vi "Data Analysis.vi"(8 "error in (no error)":errorcluster) -> (0 "error out":errorcluster)   [LabVIEW 2016, in "User Interface.lvlib"]
uses:
  User Interface.lvlib
  DAQ Hardware/Signal name Array.ctl
  DAQ Hardware/Data View Commnd.ctl
  DAQ Hardware/Data Analysis Main Cluster.ctl
  <vilib>/NI/Current Value Table/DataTypes/Array of Double_Read.vi
  <vilib>/NI/Current Value Table/DataTypes/Single_Read.vi
  <vilib>/NI/Current Value Table/DataTypes/Boolean_Read.vi
  <vilib>/NI/Current Value Table/Type to Enum.vi
  <vilib>/NI/Current Value Table/DataTypes/Array of Double_Type To Enum.vi
  <vilib>/NI/Current Value Table/DataTypes/Single_Type To Enum.vi
  <vilib>/NI/Current Value Table/DataTypes/Boolean_Type To Enum.vi
  <vilib>/NI/Current Value Table/FGVs/Group Memory.vi
  <vilib>/NI/Current Value Table/FGVs/Tag Memory.vi
  <vilib>/NI/Current Value Table/FGVs/CVT Globals.vi
  <vilib>/NI/Current Value Table/Memory Block.vi
  <vilib>/NI/Current Value Table/DataTypes/Array of Double_Memory Block.vi
  <vilib>/NI/Current Value Table/DataTypes/Single_Memory Block.vi
  <vilib>/NI/Current Value Table/DataTypes/Boolean_Memory Block.vi
  DAQ Hardware/DAQ Hardware.lvlib
  <vilib>/NI/Current Value Table/Current Value Table.lvlib
panel:
  out "Time":string="Sat  8/3/2019  8:10:44 PM"
  in  "Exit":bool
  out "Analog Data":dbl[][](graph)
  in  "Signal Selection":T1=[{"Select"=FALSE, "Signal name"=""}, {"Select"=FALSE, "Signal name"=""}, {"Select"=FALSE, "Signal name"=""}, {"Select"=FALSE, "Signal name"=""}]
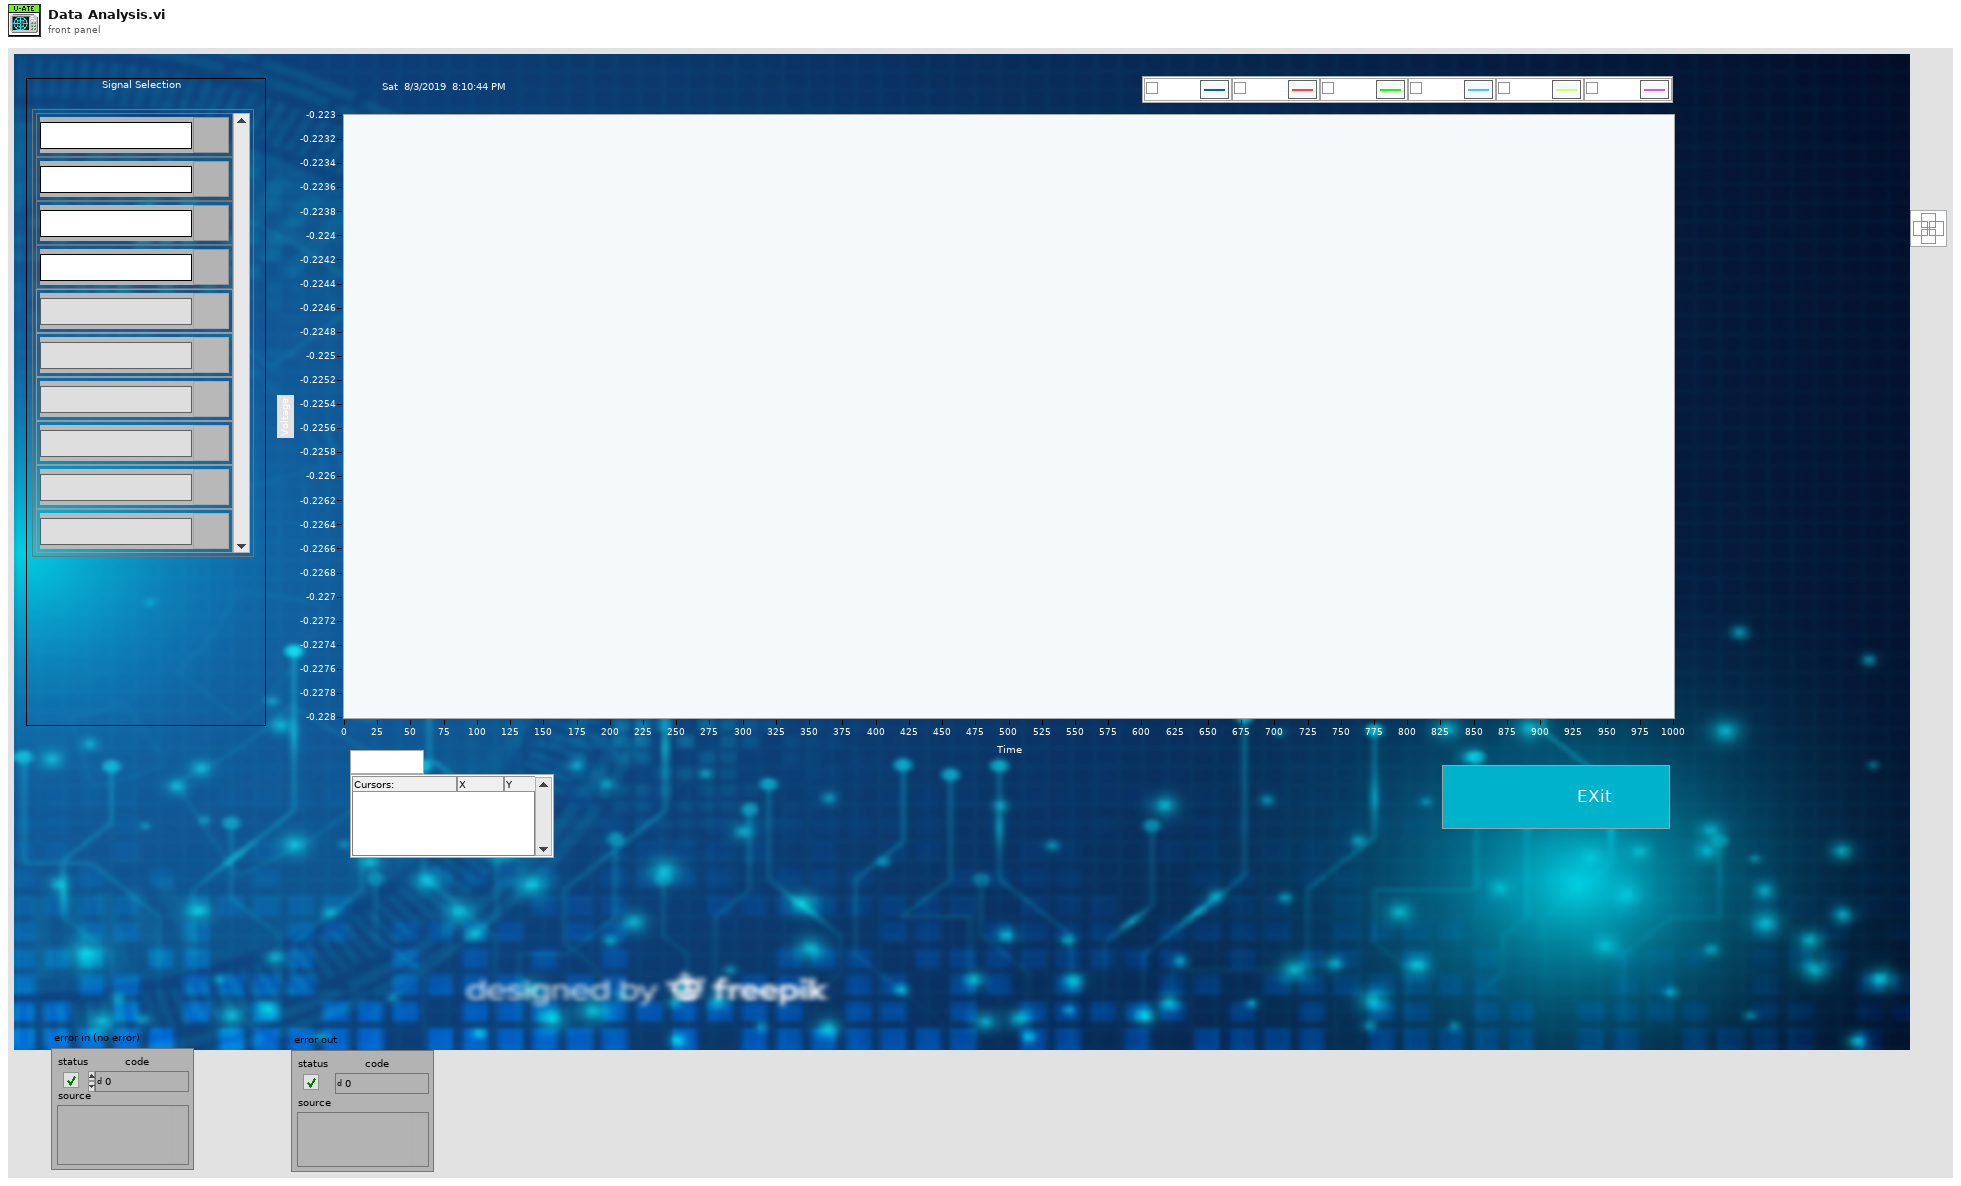
[diagram p1: front panel]
types:
  T1 = typedef "DAQ Hardware.lvlib/Signal name Array.ctl" = cluster{"Select":bool, "Signal name":string}[]
  T2 = typedef "DAQ Hardware.lvlib/Data Analysis Main Cluster.ctl" = cluster{"Active Signal":cluster{"Select":bool, "Signal name":string}[]}
  T3 = typedef "DAQ Hardware.lvlib/Data View Commnd.ctl" = enum16{"Init", "Main", "Close"}
  T4 = typedef "CVT.lvlib/Current Value Table.lvlib/Data Types.ctl" = enum16{"Double", "Single", "I64", "I32", "I16", "I8", "U64", "U32", "U16", "U8", "String", "Boolean", "Array of U8", "Array of U16", "Array of U32", "Array of U64", "Array of I64", "Array of I32", "Array of I16", "Array of I8", "Array of Double", "Array of Single", "Array of Boolean", "Array of String"}
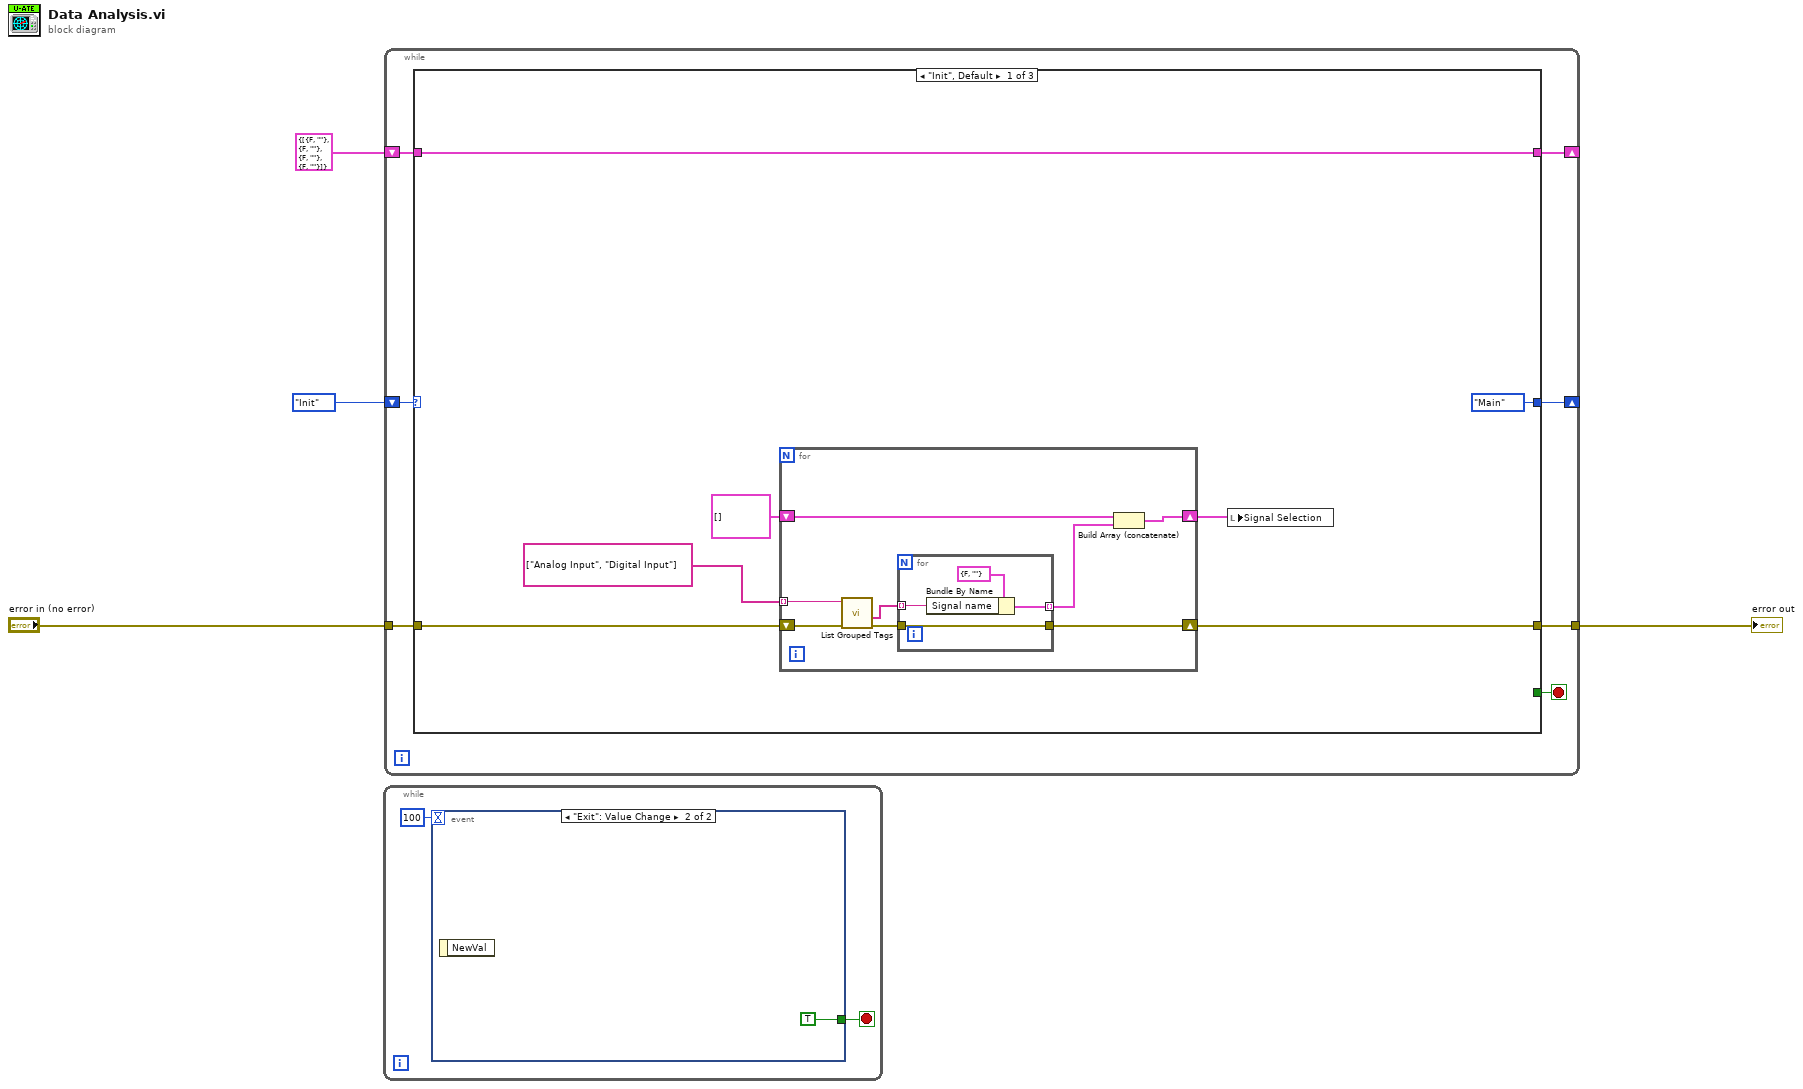
[diagram p0: block diagram]
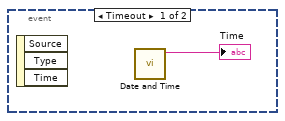
[diagram p2: hidden frame]
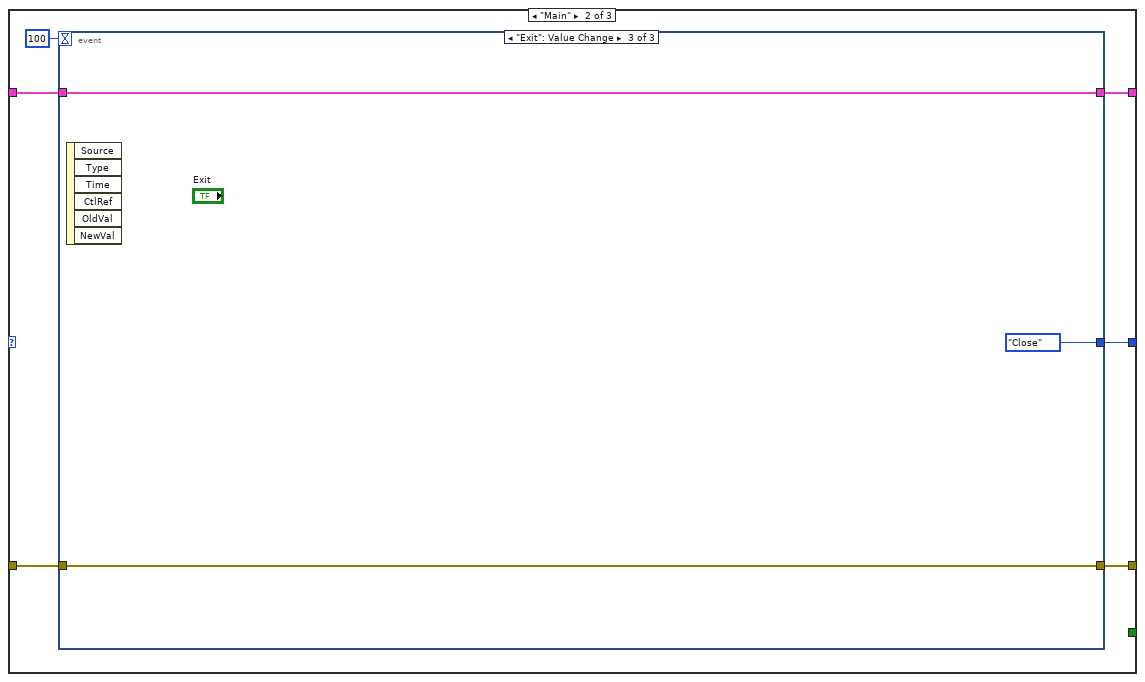
[diagram p3: hidden frame]
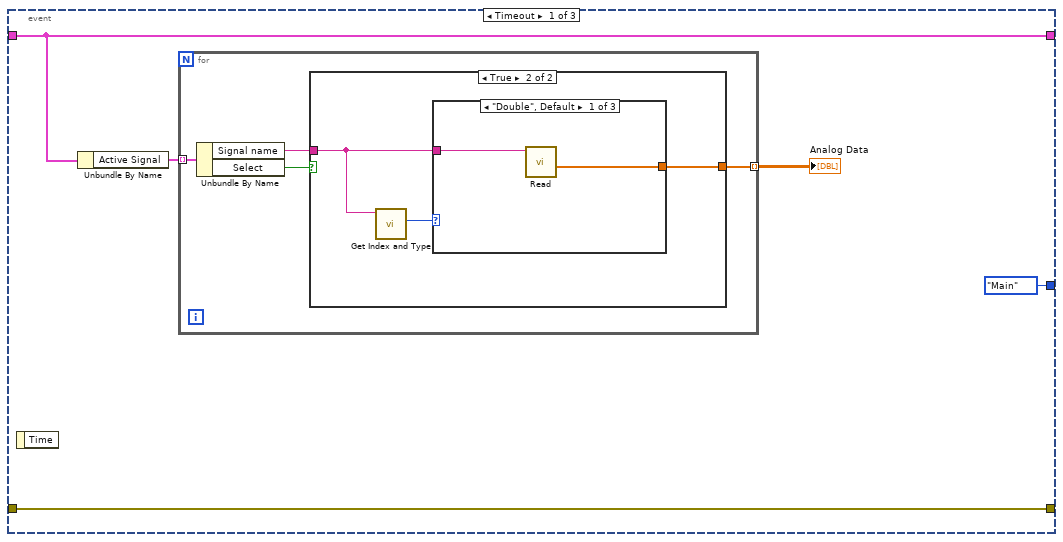
[diagram p4: hidden frame]
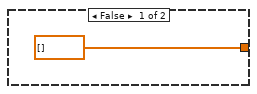
[diagram p5: hidden frame]
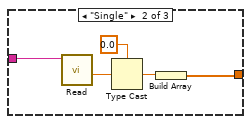
[diagram p6: hidden frame]
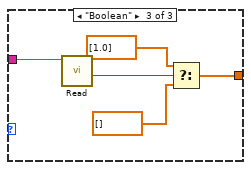
[diagram p7: hidden frame]
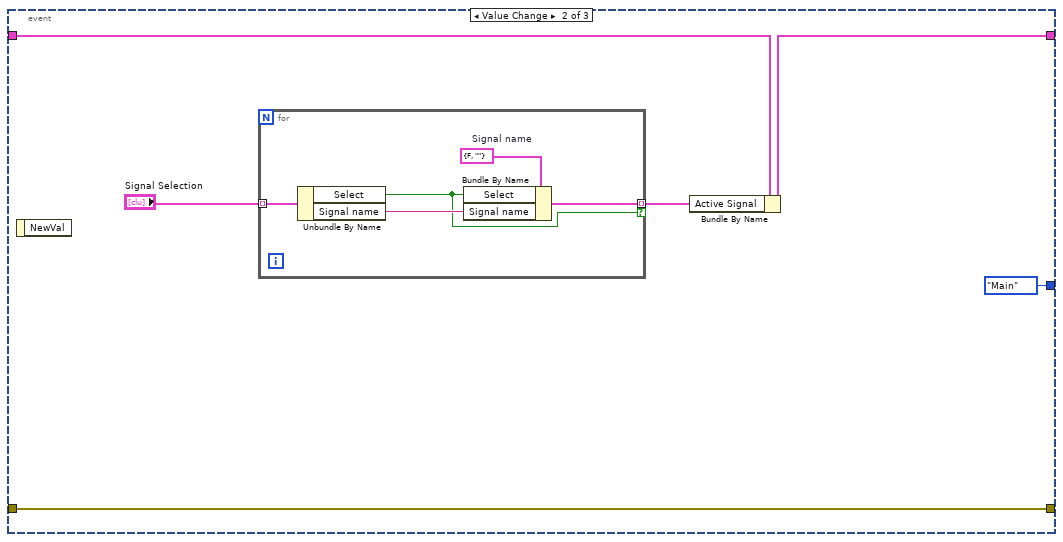
[diagram p8: hidden frame]
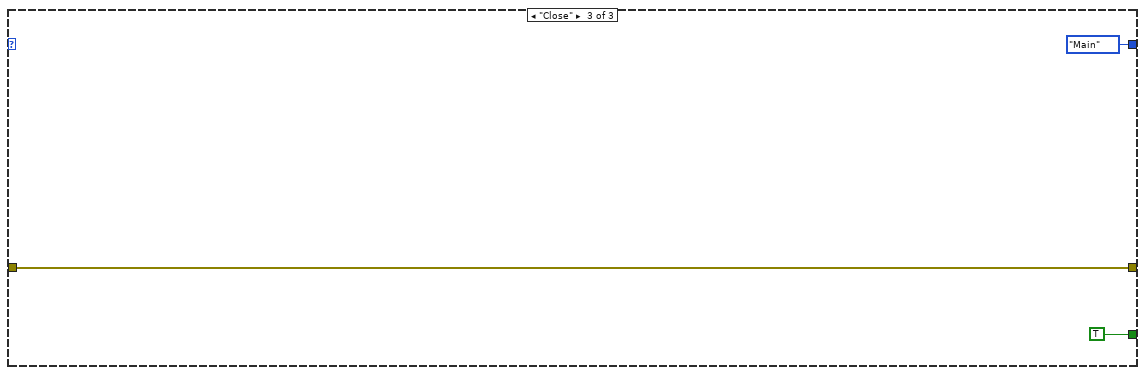
[diagram p9: hidden frame]
diagram:
  n1 = while {
    stop <- w5 stop-if-true
    n2 = event shown="[1] \"Exit\": Value Change" {
      selector: _ -> [_ _]
      dyn-events: _ -> [_ _]
      timeout: 100 -> [_ _]
      tunnel: [_ TRUE] -> w5
      event Timeout {
        n3 = event-data() -> ()  [unwired: 1 in, 3 out]
        n4 = call "Date and Time.vi"() -> ("Current Time"=→"Time":string)  [unwired: 11 in]
      }
      event "Exit": Value Change {
        n5 = event-data() -> ()  [unwired: 1 in, 1 out]
      }
    }
  }
  n6 = while {
    shift-right: [w15] -> _
    shift-left: Data_View_Commnd."Init" -> [w9]
    tunnel: "error in (no error)" -> [w13]
    tunnel: [w12] -> w3
    shift-right: [w10] -> _
    shift-left: T2 {"Active Signal"=[{"Select"=FALSE, "Signal name"=""}, {"Select"=FALSE, "Signal name"=""}, {"Select"=FALSE, "Signal name"=""}, {"Select"=FALSE, "Signal name"=""}]} -> [w11]
    stop <- w14 stop-if-true
    n7 = case shown="\"Init\", Default" w9 {
      tunnel: [Data_View_Commnd."Main" w40 Data_View_Commnd."Main"] -> w15
      tunnel: [_ _ TRUE] -> w14
      tunnel: w13 -> [w17 w39 w80]
      tunnel: [w16 w38 w80] -> w12
      tunnel: w11 -> [w21 w37 _]
      tunnel: [w21 w36 _] -> w10
      frame "Init", Default {
        n8 = for {
          shift-right: [w26] -> w16
          shift-left: w17 -> [w30]
          tunnel: string[] ["Analog Input", "Digital Input"] -> [w25] mode=indexing
          shift-right: [w24] -> w20
          shift-left: cluster{"Select":bool, "Signal name":string}[] [] -> [w23]
          n9 = call <vilib>:"List Grouped Tags.vi"("error in (no error)"=w30, "Group"=w25) -> ("error out"=w29:errorcluster, "Tags Out"=w28:string[])  [unwired: 8 in]
          n10 = for {
            tunnel: w29 -> [w32]
            tunnel: w28 -> [w33] mode=indexing
            tunnel: [w32] -> w26
            tunnel: [w31] -> w27 mode=indexing
            n11 = Bundle By Name(cluster=cluster{"Select":bool, "Signal name":string} {"Select"=FALSE, "Signal name"=""} ("Cluster"), "Signal name"=w33) -> (w31:cluster{"Select":bool, "Signal name":string})
          }
          n12 = Build Array (concatenate)(w23, w27) -> (w24:cluster{"Select":bool, "Signal name":string}[])
        }
        n13 = local write "Signal Selection"(w20) -> ()
      }
      frame "Main" {
        n14 = event shown="[2] \"Exit\": Value Change" {
          selector: _ -> [_ _ _]
          dyn-events: _ -> [_ _ _]
          timeout: 100 -> [_ _ _]
          tunnel: [Data_View_Commnd."Main" Data_View_Commnd."Main" Data_View_Commnd."Close"] -> w40
          tunnel: w39 -> [w43 w71 w77]
          tunnel: [w43 w71 w77] -> w38
          tunnel: w37 -> [w44 w69 w78]
          tunnel: [w44 w67 w78] -> w36
          event Timeout {
            n15 = event-data() -> ()  [unwired: 1 in, 1 out]
            n16 = Unbundle By Name(w44) -> ("Active Signal"=w42:cluster{"Select":bool, "Signal name":string}[])
            n17 = for {
              tunnel: w42 -> [w49] mode=indexing
              tunnel: [w47] -> w41 mode=indexing
              n18 = Unbundle By Name(w49) -> ("Signal name"=w48:string, "Select"=w46:bool)
              n19 = case shown="True" w46 {
                tunnel: w48 -> [_ w52]
                tunnel: [dbl[] [] ("Value") w53] -> w47
                frame False {
                }
                frame True {
                  n20 = call <vilib>:"Get Index and Type.vi"("Tag"=w52) -> ("Type"=w51:T4)  [unwired: 8 in, 2 out]
                  n21 = case shown="\"Double\", Default" w51 {
                    tunnel: [w55 w56 w62] -> w53
                    tunnel: w52 -> [w54 w60 w65]
                    frame "Double", Default {
                      n22 = call-poly <vilib>:"Read.vi"("Tag Name"=w54) -> ("Value"=w55:dbl[])  [unwired: 9 in, 1 out]
                    }
                    frame "Single" {
                      n23 = call-poly <vilib>:"Read.vi"("Tag Name"=w60) -> ("Value"=w59:sgl)  [unwired: 9 in, 1 out]
                      n24 = Type Cast(type=0.0 ("Value"), x=w59) -> (*(type *) &x=w57:dbl)
                      n25 = Build Array(w57) -> (w56:dbl[])
                    }
                    frame "Boolean" {
                      n26 = call-poly <vilib>:"Read.vi"("Tag Name"=w65) -> ("Value"=w64:bool)  [unwired: 9 in, 1 out]
                      n27 = Select(t=dbl[] [1.0] ("Value"), s=w64, f=dbl[] [] ("Value")) -> (s? t:f=w62:dbl[])
                    }
                  }
                }
              }
            }
            "Analog Data" <- w41
          }
          event Value Change {
            n28 = event-data() -> ()  [unwired: 1 in, 1 out]
            n29 = for {
              tunnel: "Signal Selection" -> [w76] mode=indexing
              tunnel: [w74] -> w66 mode=indexing if=w72
              w73 = cluster{"Select":bool, "Signal name":string} {"Select"=FALSE, "Signal name"=""}  # Signal name
              n30 = Unbundle By Name(w76) -> ("Select"=w72:bool, "Signal name"=w75:string)
              n31 = Bundle By Name(cluster=w73, "Select"=w72, "Signal name"=w75) -> (w74:cluster{"Select":bool, "Signal name":string})
            }
            n32 = Bundle By Name(cluster=w69, "Active Signal"=w66) -> (w67:T2)
          }
          event "Exit": Value Change {
            n33 = event-data() -> ()  [unwired: 1 in, 6 out]
          }
        }
      }
      frame "Close" {
      }
    }
  }
  "error out" <- w3
